vi "Teleop.vi"(10 "Match Info":T1={"Autonomous Elapsed Seconds"=0.0, "TeleOp Elapsed Seconds"=0.0, "Disabled Elapsed Seconds"=0.0, "Visited Autonomous"=FALSE, "Visited TeleOp"=FALSE, "Visited Disabled"=FALSE, "Autonomous Settings"={"Autonomous Style"=enum."Independent", "VI Refnum"=refnum}}, 11 "Call Context":T2) -> ()   [LabVIEW 2019]
doc: "This VI is called for each enabled TeleOp packet received from the DS. It is typically used to read from joysticks and other inputs and update I/O or setpoints for timed control loops. It should complete and return within 20 milliseconds or risk missing DS packets."
uses:
  <vilib>/Rock Robotics/WPI/DriverStation/WPI_DriverStationDerivedRobotMode.ctl
  <vilib>/Rock Robotics/WPI/DriverStation/WPI_DriverStationMatch Info.ctl
  Upper Transfer/Implementation/Upper Transfer Operations.ctl
  <vilib>/Rock Robotics/WPI/Utilities/WPI_GetSetVariantRefNum.vi
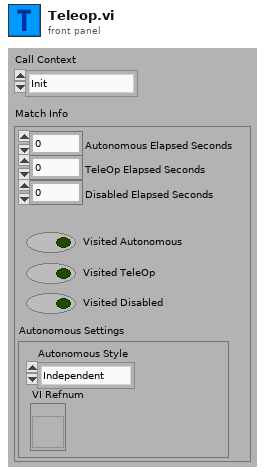
[diagram p1: front panel]
types:
  T1 = typedef "WPI_DriverStationMatch Info.ctl" = cluster{"Autonomous Elapsed Seconds":dbl, "TeleOp Elapsed Seconds":dbl, "Disabled Elapsed Seconds":dbl, "Visited Autonomous":bool, "Visited TeleOp":bool, "Visited Disabled":bool, "Autonomous Settings":cluster{"Autonomous Style":enum16{"Iterative", "Independent"}, "VI Refnum":refnum<vi>}}
  T2 = typedef "WPI_DriverStationDerivedRobotMode.ctl" = enum16{"Init", "Execute", "Stop"}
  T3 = typedef "Upper Transfer Operations.ctl" = enum16{"Reserve", "Read Current", "Immediate"}
  T4 = typedef "WPI_JoystickDevRef.ctl" = cluster{"Device":T5}
  T5 = typedef "WPI_JoystickDeviceEnum.ctl" = enum16{"USB 0", "USB 1", "USB 2", "USB 3", "USB 4", "USB 5"}
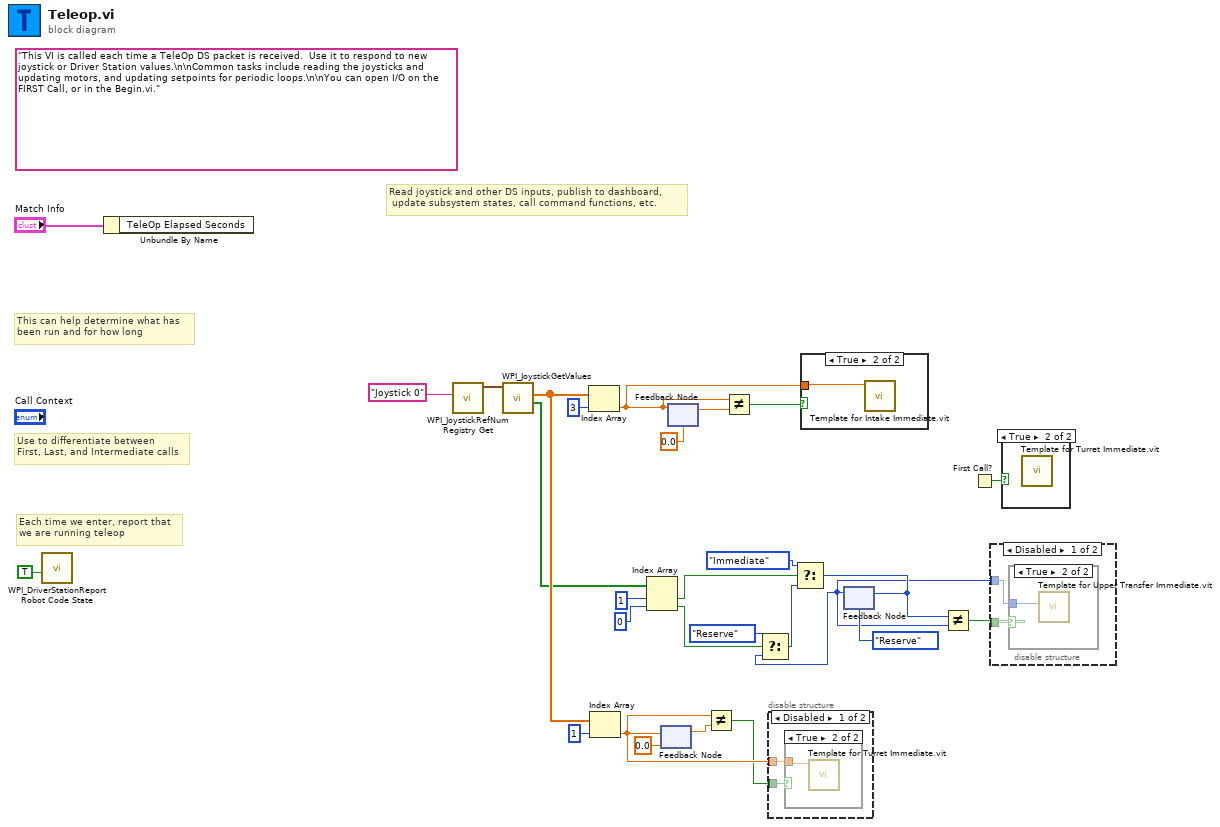
[diagram p0: block diagram]
diagram:
  (unwired) "This VI is called each time a TeleOp DS packet is received.  Use it to respond to new joystick or Driver Station values.\n\nCommon tasks include reading the joysticks and updating motors, and updating setpoints for periodic loops.\n\nYou can open I/O on the FIRST Call, or in the Begin.vi."
  # "Read joystick and other DS inputs, publish to dashboard,\n update subsystem states, call command functions, etc."
  # "Each time we enter, report that\nwe are running teleop"
  # "Use to differentiate between\nFirst, Last, and Intermediate calls"
  # "This can help determine what has\nbeen run and for how long"
  n1 = call <vilib>:"WPI_DriverStationReport Robot Code State.vi"("TeleOp"=TRUE ("Autonomous")) -> ()  [unwired: 10 in, 1 out]
  n2 = Unbundle By Name("Match Info") -> ()  [unwired: 1 out]
  n3 = call <vilib>:"WPI_JoystickRefNum Registry Get.vi"("refnum name"="Joystick 0") -> ("JoystickDevRef"=w25:T4)  [unwired: 1 in, 9 out]
  n4 = call <vilib>:"WPI_JoystickGetValues.vi"("JoystickDevRef"=w25) -> ("Buttons"=w13:bool[], "Axes"=w20:dbl[])  [unwired: 6 in, 3 out]
  n5 = Index Array(array=w20, index=3) -> (element=w15:dbl)
  n6 = Index Array(array=w20, index=1) -> (element=w14:dbl)
  n7 = Index Array(array=w13, index #1=1 ("index"), index #2=0 ("index")) -> (element #1=w11:bool, element #2=w10:bool)
  n8 = feedback #1(0.0 ("upper limit")) -> (w17:dbl)
  n9 = feedback-in #1(w14) -> ()
  n10 = feedback-in #2(w15) -> ()
  n11 = feedback #2(0.0 ("upper limit")) -> (w22:dbl)
  n12 = Not Equal?(x=w14, y=w17) -> (x != y?=w2:bool)
  n13 = Not Equal?(x=w15, y=w22) -> (x != y?=w16:bool)
  n14 = disable-structure shown="Disabled" {
    disable-tunnel: w14 -> [w30 _]
    disable-tunnel: w2 -> [w29 _]
    frame Disabled {
      n15 = case shown="True" w29 {
        tunnel: w30 -> [_ w31]
        frame False {
        }
        frame True {
          n16 = call "Template for Turret Immediate.vit"("Power"=w31) -> ()  [unwired: 10 in, 1 out]
        }
      }
    }
    frame Enabled {
    }
  }
  n17 = case shown="True" w16 {
    tunnel: w15 -> [_ w32]
    frame False {
    }
    frame True {
      n18 = call "Template for Intake Immediate.vit"("Power"=w32) -> ()  [unwired: 10 in, 1 out]
    }
  }
  n19 = feedback #3(Upper_Transfer_Operations."Reserve" ("Operation")) -> (w4:T3)
  n20 = Select(t=Upper_Transfer_Operations."Reserve" ("Operation"), s=w10, f=w4) -> (s? t:f=w9:T3)
  n21 = Select(t=Upper_Transfer_Operations."Immediate" ("Operation"), s=w11, f=w9) -> (s? t:f=w5:T3)
  n22 = feedback-in #3(w5) -> ()
  n23 = Not Equal?(x=w5, y=w4) -> (x != y?=w6:bool)
  n24 = First Call?() -> (First Call?: T/F=w1:bool)
  n25 = disable-structure shown="Disabled" {
    disable-tunnel: w6 -> [w34 _]
    disable-tunnel: w4 -> [w33 _]
    frame Disabled {
      n26 = case shown="True" w34 {
        tunnel: w33 -> [_ w35]
        frame False {
        }
        frame True {
          n27 = call "Template for Upper Transfer Immediate.vit"("Operation"=w35) -> ()  [unwired: 10 in, 1 out]
        }
      }
    }
    frame Enabled {
    }
  }
  n28 = case shown="True" w1 {
    frame False {
    }
    frame True {
      n29 = call "Template for Turret Immediate.vit"() -> ()  [unwired: 11 in, 1 out]
    }
  }
